vi "MACBIN Encode MacBinary__ogtk.vi"(4 "error in (no error)":errorcluster, 5 "macbinary file":path, 6 "resource file":path, 7 "data file":path) -> (0 "error out":errorcluster, 1 "macbinary file out":path, 2 "resource file out":path, 3 "data file out":path)   [LabVIEW 2012]
doc: "Encodes a Macintosh File to MacBinary format."
uses:
  <userlib>/_OpenG.lib/file/file.llb/Valid Path - Traditional__ogtk.vi
panel:
  # "Please visit http://www.OpenG.org to learn about the\nOpen Source LabVIEW software movement.\n\nNOTICE -- YOU MUST LEAVE THIS NOTICE IN PLACE.  PER THE TERMS OF THE LICENSE BELOW, YOU MAY SUBLICENSE THIS SOFTWARE \nIN ANY WAY THAT DOES NOT CONFLICT WITH THIS LICENSE.\n\n### BSD License (http://www.opensource.org/licenses/bsd-license.php) Begin ###\n \nCopyright (C) 2002 Christophe Salzmann christophe.salzmann@epfl.ch\nCopyright (C) 2002-2006 Rolf Kalbermatter rolf.kalbermatter@citengineering.com\n\nAll rights reserved.\n\nRedistribution and use in source and binary forms, with or without modification, are permitted provided that the following conditions are met:\n\n    * Redistributions of source code must retain the above copyright notice, this list of conditions and the following disclaimer.\n    * Redistributions in binary form must reproduce the above copyright notice, this list of conditions and the following disclaimer in the \n       documentation and/or other materials provided with the distribution.\n    * Neither the name of SciWare, James Kring, Inc., nor the names of its contributors may be used to endorse or promote products derived \n       from this software without specific prior written permission.\n\nTHIS SOFTWARE IS PROVIDED BY THE COPYRIGHT HOLDERS AND CONTRIBUTORS \"AS IS\" AND ANY EXPRESS OR IMPLIED WARRANTIES, \nINCLUDING, BUT NOT LIMITED TO, THE IMPLIED WARRANTIES OF MERCHANTABILITY AND FITNESS FOR A PARTICULAR PURPOSE ARE \nDISCLAIMED. IN NO EVENT SHALL THE COPYRIGHT OWNER OR CONTRIBUTORS BE LIABLE FOR ANY DIRECT, INDIRECT, INCIDENTAL,\n SPECIAL, EXEMPLARY, OR CONSEQUENTIAL DAMAGES (INCLUDING, BUT NOT LIMITED TO, PROCUREMENT OF SUBSTITUTE GOODS OR \nSERVICES; LOSS OF USE, DATA, OR PROFITS; OR BUSINESS INTERRUPTION) HOWEVER CAUSED AND ON ANY THEORY OF LIABILITY, \nWHETHER IN CONTRACT, STRICT LIABILITY, OR TORT (INCLUDING NEGLIGENCE OR OTHERWISE) ARISING IN ANY WAY OUT OF THE USE \nOF THIS SOFTWARE, EVEN IF ADVISED OF THE POSSIBILITY OF SUCH DAMAGE.\n\n### BSD License End ###"
  # "``"
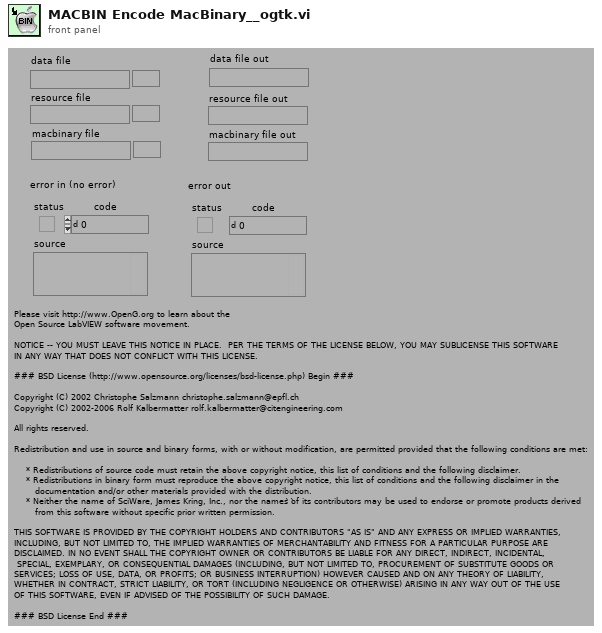
[diagram p1: front panel]
types:
  T1 = enum16{"open", "replace", "create", "open or create", "replace or create", "replace or create with confirmation"}
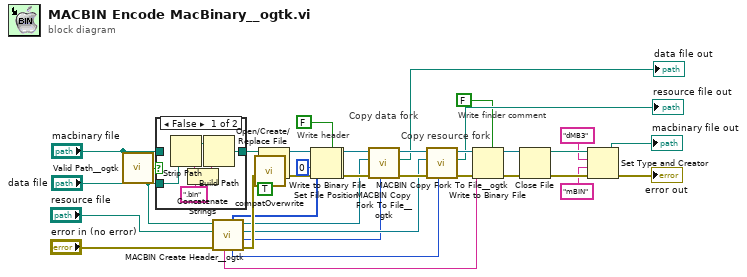
[diagram p0: block diagram]
diagram:
  # "Write header"
  # "Write finder comment"
  # "Copy resource fork"
  # "Copy data fork"
  n1 = call-poly <userlib>:"Valid Path__ogtk.vi"("path"="macbinary file") -> ("valid"=w16:bool)
  n2 = case shown="False" w16 {
    tunnel: "macbinary file" -> [_ w45]
    tunnel: [w43 w45] -> w14
    tunnel: "data file" -> [w44 _]
    frame False {
      n3 = Strip Path(path=w44) -> (stripped path=w42:path, name=w41:string)
      n4 = Concatenate Strings(w41, ".bin" ("Substring")) -> (w40:string)
      n5 = Build Path(base path=w42, name or relative path=w40) -> (appended path=w43:path)
    }
    frame True {
    }
  }
  n6 = call <userlib>:"MACBIN Create Header__ogtk.vi"("data file"="data file", "resource file"="resource file", "error in (no error)"="error in (no error)") -> ("comment"=w30:string, "header"=w22:u8[], "res size"=w17:i32, "data refnum"=w21:refnum<file>, "res refnum"=w20:refnum<file>, "data size"=w18:i32, "error out"=w28:errorcluster)  [unwired: 1 in]
  n7 = call <vilib>:"compatOverwrite.vi"("overwrite (F)"=TRUE) -> ("overwrite?"=w1:T1)
  n8 = Open/Create/Replace File(file path (use dialog)=w14, error in=w28, operation (0:open)=w1) -> (refnum out=w38:refnum<file>, error out=w37:errorcluster)  [unwired: 3 in, 1 out]
  n9 = Set File Position(offset (in bytes) (0)=0 ("pos offset (0)"), refnum=w38, error in=w37) -> (refnum out=w4:refnum<file>, error out=w3:errorcluster)  [unwired: 1 in]
  n10 = Write to Binary File(file (use dialog)=w4, data=w22, error in=w3, 5:FALSE ("prepend array or string size? (T)")) -> (refnum out=w34:refnum<file>, error out=w29:errorcluster)  [unwired: 2 in, 1 out]
  n11 = call <userlib>:"MACBIN Copy Fork To File__ogtk.vi"("file size"=w18, "error out"=w29, "fork Refnum"=w21, "macbinary Refnum"=w34) -> ("error out"=w27:errorcluster, "filename out"=→"data file out":path, "macbinary Refnum out"=w26:refnum<file>)  [unwired: 2 in]
  n12 = call <userlib>:"MACBIN Copy Fork To File__ogtk.vi"("file size"=w17, "error out"=w27, "fork Refnum"=w20, "macbinary Refnum"=w26) -> ("error out"=w25:errorcluster, "filename out"=→"resource file out":path, "macbinary Refnum out"=w24:refnum<file>)  [unwired: 2 in]
  n13 = Write to Binary File(file (use dialog)=w24, data=w30, error in=w25, 5:FALSE ("prepend array or string size? (T)")) -> (refnum out=w32:refnum<file>, error out=w31:errorcluster)  [unwired: 2 in, 1 out]
  n14 = Close File(refnum=w32, error in=w31) -> (path=w8:path, error out=w10:errorcluster)
  n15 = Set Type and Creator(4:w10, 5:"mBIN" ("new creator"), 6:"dMB3" ("new type"), 7:w8) -> (0:→"error out":errorcluster, 3:→"macbinary file out":path)
